vi "Create.vi"   [LabVIEW 2020, in "image.lvlib" / "Image to File-Buffer Encoder.lvclass"]
uses:
  Image to File-Buffer Encoder.lvclass
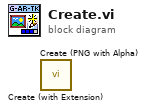
[diagram p0: block diagram]
diagram:
  n1 = call "Create (with Extension).vi"() -> ()  [unwired: 10 in, 2 out]
  n2 = call "Create (PNG with Alpha).vi"() -> ()  [unwired: 10 in, 2 out]
